vi "geve-msg_enqueue_at_opposite_end.vi"(8 "error in (no error)":errorcluster, 10 "Message":T1, 11 "Runtime Data":T2) -> (0 "error out":errorcluster)   [LabVIEW 2018]
doc: "enqueuer at opposite end for the worker loop"
uses:
  geve-runtime_data_cluster.ctl
  geve-monitoring_data_cluster.ctl
  geve-serial_config_cluster.ctl
  geve-com_ref_cluster.ctl
  geve-message_cluster.ctl
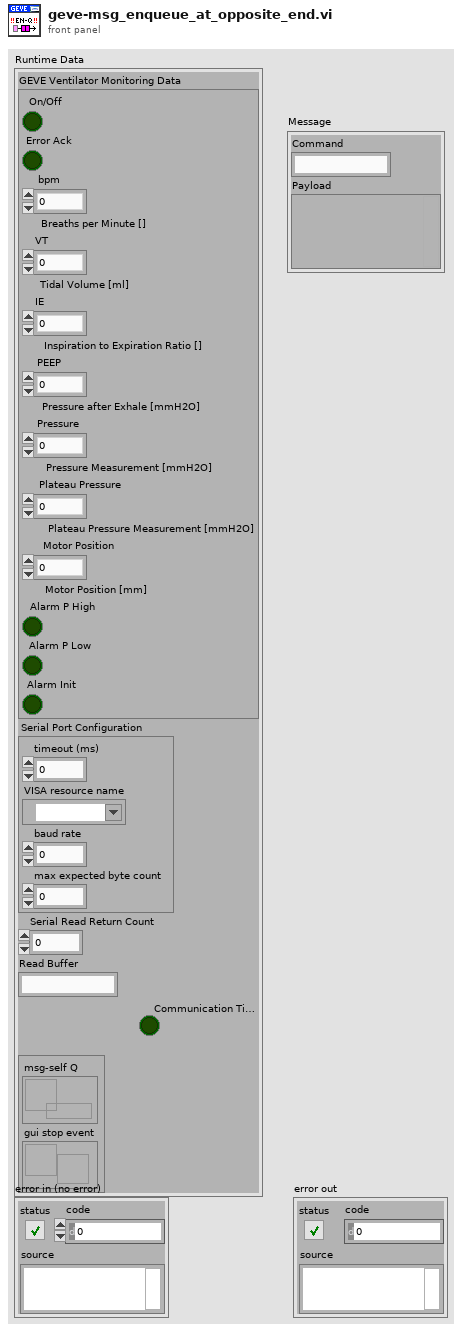
[diagram p1: front panel]
types:
  T1 = typedef "geve-message_cluster.ctl" = cluster{"Command":string, "Payload":variant}
  T2 = typedef "geve-runtime_data_cluster.ctl" = cluster{"GEVE Ventilator Monitoring Data":T3, "Serial Port Configuration":T4, "Serial Read Return Count":u32, "Read Buffer":string, "Communication Timeout?":bool, "com-refs":T5}
  T3 = typedef "geve-monitoring_data_cluster.ctl" = cluster{"On/Off":bool, "Error Ack":bool, "bpm":dbl, "VT":dbl, "IE":dbl, "PEEP":dbl, "Pressure":dbl, "Plateau Pressure":dbl, "Motor Position":dbl, "Alarm P High":bool, "Alarm P Low":bool, "Alarm Init":bool}
  T4 = typedef "geve-serial_config_cluster.ctl" = cluster{"timeout (ms)":u32, "VISA resource name":refnum<visa-resource-name>, "baud rate":u32, "max expected byte count":u32}
  T5 = typedef "geve-com_ref_cluster.ctl" = cluster{"msg-self Q":refnum<queue>, "gui stop event":refnum<user-event>}
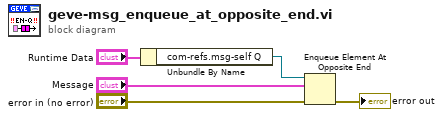
[diagram p0: block diagram]
diagram:
  n1 = Unbundle By Name("Runtime Data") -> ("com-refs.msg-self Q"=w5:refnum<queue>)
  n2 = Enqueue Element At Opposite End(queue=w5, element="Message", error in (no error)="error in (no error)") -> (error out=→"error out":errorcluster)  [unwired: 1 in, 2 out]
